vi "WriteGroupedDigitalOutputs.vi"(8 "error in (no error)":errorcluster, 10 "data":u32, 11 "TesteractHAL_DigitalOutput_NIDAQmx In":refnum<class "TesteractHAL_DigitalOutput_NIDAQmx.lvclass">) -> (0 "error out":errorcluster, 3 "TesteractHAL_DigitalOutput_NIDAQmx Out":refnum<class "TesteractHAL_DigitalOutput_NIDAQmx.lvclass">)   [LabVIEW 2017, in "TesteractHAL_DigitalOutput_NIDAQmx.lvlib" / "TesteractHAL_DigitalOutput_NIDAQmx.lvclass"]
doc: "Write a U32 value to the port that the device based on."
uses:
  TesteractHAL_DigitalOutput_NIDAQmx.lvclass
  TesteractHAL_DigitalOutput_NIDAQmx.lvclass/TesteractHAL_DigitalOutput_NIDAQmx.ctl
  <vilib>/DAQmx/write.llb/DAQmx Write (Digital U32 1Chan 1Samp).vi
  <vilib>/DAQmx/miscellaneous.llb/DAQmx Fill In Error Info.vi
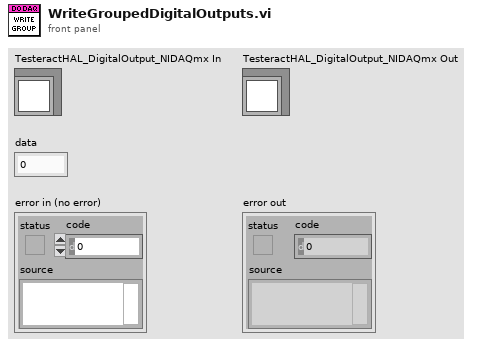
[diagram p1: front panel]
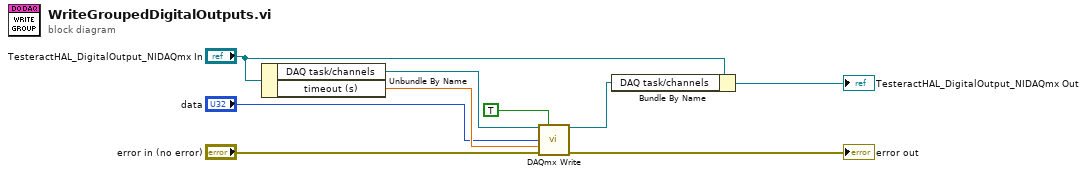
[diagram p0: block diagram]
diagram:
  n1 = Unbundle By Name("TesteractHAL_DigitalOutput_NIDAQmx In") -> ("DAQ task/channels"=w7:refnum<k21>, "timeout (s)"=w2:dbl)
  n2 = call-poly <vilib>:"DAQmx Write.vi"("task/channels in"=w7, "auto start"=TRUE, "data"="data", "timeout"=w2, "error in"="error in (no error)") -> ("task out"=w4:refnum<k21>, "error out"=→"error out":errorcluster)  [unwired: 8 in, 1 out]
  n3 = Bundle By Name(cluster="TesteractHAL_DigitalOutput_NIDAQmx In", "DAQ task/channels"=w4) -> (→"TesteractHAL_DigitalOutput_NIDAQmx Out":refnum<class "TesteractHAL_DigitalOutput_NIDAQmx.lvclass">)
